vi "Get Event ID.vi"(8 "error in (no error)":errorcluster, 11 "Event in":refnum<class "Event.lvclass">) -> (0 "error out":errorcluster, 2 "Event ID":string, 3 "Event out":refnum<class "Event.lvclass">)   [LabVIEW 2016, in "Event Source.lvlib" / "Event.lvclass"]
doc: "Gets the unique ID of the event specific class"
uses:
  Event.lvclass
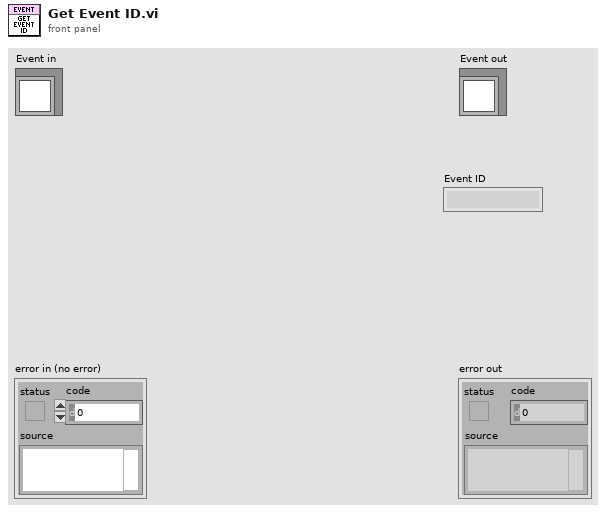
[diagram p1: front panel]
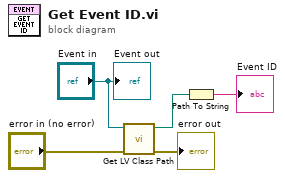
[diagram p0: block diagram]
diagram:
  n1 = call <vilib>:"Get LV Class Path.vi"("error in (no error)"="error in (no error)", "object"="Event in") -> ("error out"=→"error out":errorcluster, "class path"=w2:path)  [unwired: 8 in]
  n2 = Path To String(path=w2) -> (string=→"Event ID":string)
  "Event out" <- "Event in"
